vi "Read Instant Digital.vi"(11 "ADALM2000 Handler":u32 caption="Instrument Handle Out") -> (1 "Read value group CH 8-15":u64(slide) max=255 scale=0.0..255.0, 2 "Read value group CH 0-7":u64(slide) max=255 scale=0.0..255.0, 3 "ADALM2000 Handler 2":u32 caption="Instrument Handle Out")   [LabVIEW 2015]
uses:
  libm2k_lv.dll
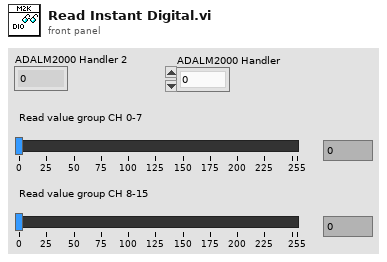
[diagram p1: front panel]
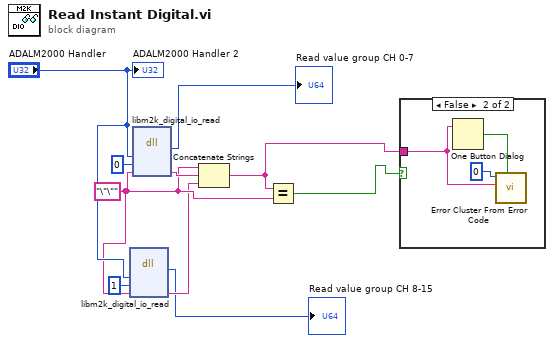
[diagram p0: block diagram]
diagram:
  w4 = "\"\""
  n1 = dll-call lib="libm2k_lv.*" fn="libm2k_digital_io_read"("instance"="ADALM2000 Handler", "groupIdx"=u64 1, "err"=w4) -> ("return type"=→"Read value group CH 8-15":u64, "err"=w3:string)  [unwired: 5 in, 2 out]
  n2 = dll-call lib="libm2k_lv.*" fn="libm2k_digital_io_read"("instance"="ADALM2000 Handler", "groupIdx"=u64 0, "err"=w4) -> ("return type"=→"Read value group CH 0-7":u64, "err"=w10:string)  [unwired: 5 in, 2 out]
  n3 = Concatenate Strings(w4, w10, w3) -> (w8:string)
  n4 = Equal?(x=w8, y=w4) -> (x = y?=w9:bool)
  n5 = case shown="False" w9 {
    tunnel: w8 -> [_ w11]
    frame True {
    }
    frame False {
      n6 = One Button Dialog(message=w11) -> (true=w13:bool)  [unwired: 1 in]
      n7 = call <vilib>:"Error Cluster From Error Code.vi"("show call chain? (False)"=w13, "error message (\"\")"=w11, "error code (0)"=0) -> ()  [unwired: 6 in, 1 out]
    }
  }
  "ADALM2000 Handler 2" <- "ADALM2000 Handler"
